vi "Handle Connections Value Change.vi"(4 "State":string, 5 "Alias Mappings":T4[](array[typedef]), 6 "Possible Connections":T3(array[cluster])=[{"Resource"="", "Possible Connections"=[]}, {"Resource"="", "Possible Connections"=[]}], 7 "Alias Mappings by Module":T1(array[cluster]), 8 "error in (no error)":errorcluster, 9 "OldVal":T5[](array[typedef]), 10 "NewVal":T5[](array[typedef]), 11 "Routing Channel Ref in":T6 format="%.0x") -> (0 "error out":errorcluster, 3 "Routing Channel Ref out":T6 format="%.0x")   [LabVIEW 2017, in "Routing and Faulting System Explorer.lvlib"]
uses:
  Routing and Faulting System Explorer.lvlib
  <vilib>/NI Veristand/Custom Device API/Custom Device Item Ref.ctl
  Connection Row.ctl
  Shared/Alias Mapping.ctl
  Shared/Routing and Faulting Hardware API/Types/Possible Connections for Endpoint.ctl
  e32bcdcd-e61b-4a24-afe7-32b08c6141fc.vi
  Scripting/Routing and Faulting Scripting.lvlib
  <vilib>/NI VeriStand/Custom Device API/Custom Device API.lvlib
  Shared/Routing and Faulting Shared.lvlib
  Shared/Routing and Faulting Hardware API/Routing and Faulting Hardware API.lvlib
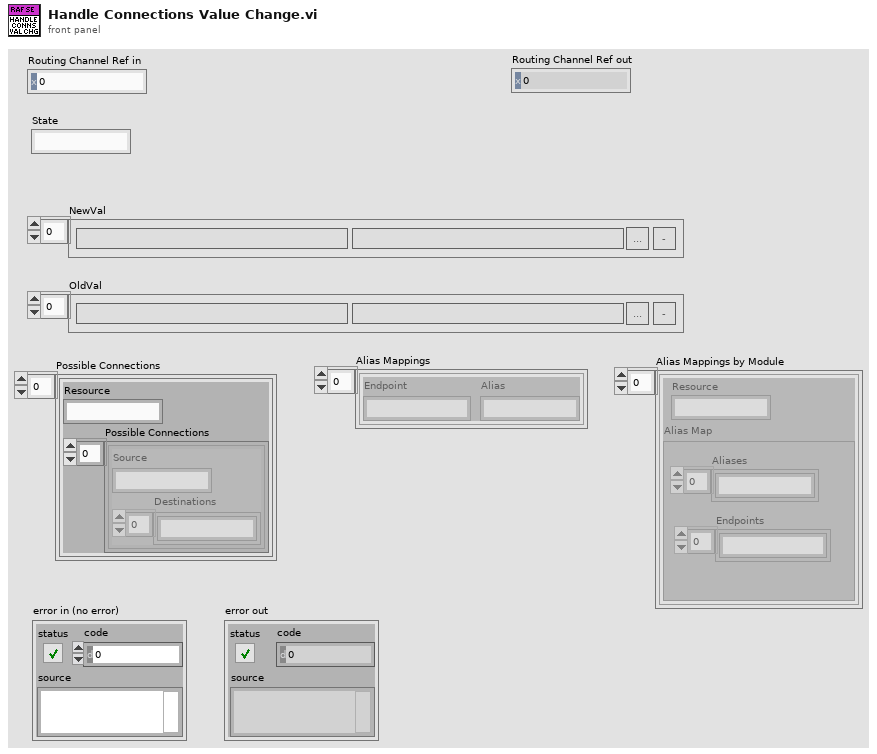
[diagram p1: front panel]
types:
  T1 = cluster{"Resource":string, "Alias Map":cluster{"Aliases":string[], "Endpoints":string[]}}[]
  T2 = typedef "Routing and Faulting Hardware API.lvlib/Possible Connections for Endpoint.ctl" = cluster{"Source":string, "Destinations":string[]}
  T3 = cluster{"Resource":string, "Possible Connections":T2[]}[]
  T4 = typedef "Routing and Faulting Shared.lvlib/Alias Mapping.ctl" = cluster{"Endpoint":string, "Alias":string}
  T5 = typedef "Routing and Faulting System Explorer.lvlib/Connection Row.ctl" = cluster{"Source":string, "Destination":string, "Edit":bool, "Remove":bool}
  T6 = typedef "Custom Device API.lvlib/Custom Device Item Ref.ctl" = u64
  T7 = cluster{"Source":bool, "Destination":bool, "Edit":bool, "Remove":bool}
  T8 = typedef "Routing and Faulting Shared.lvlib/Connection.ctl" = cluster{"Module":string, "Source":string, "Destination":string}
  T9 = typedef "Routing and Faulting Shared.lvlib/Routing State.ctl" = cluster{"Name":string, "Description":string, "Value":i32, "Connection List":T8[]}
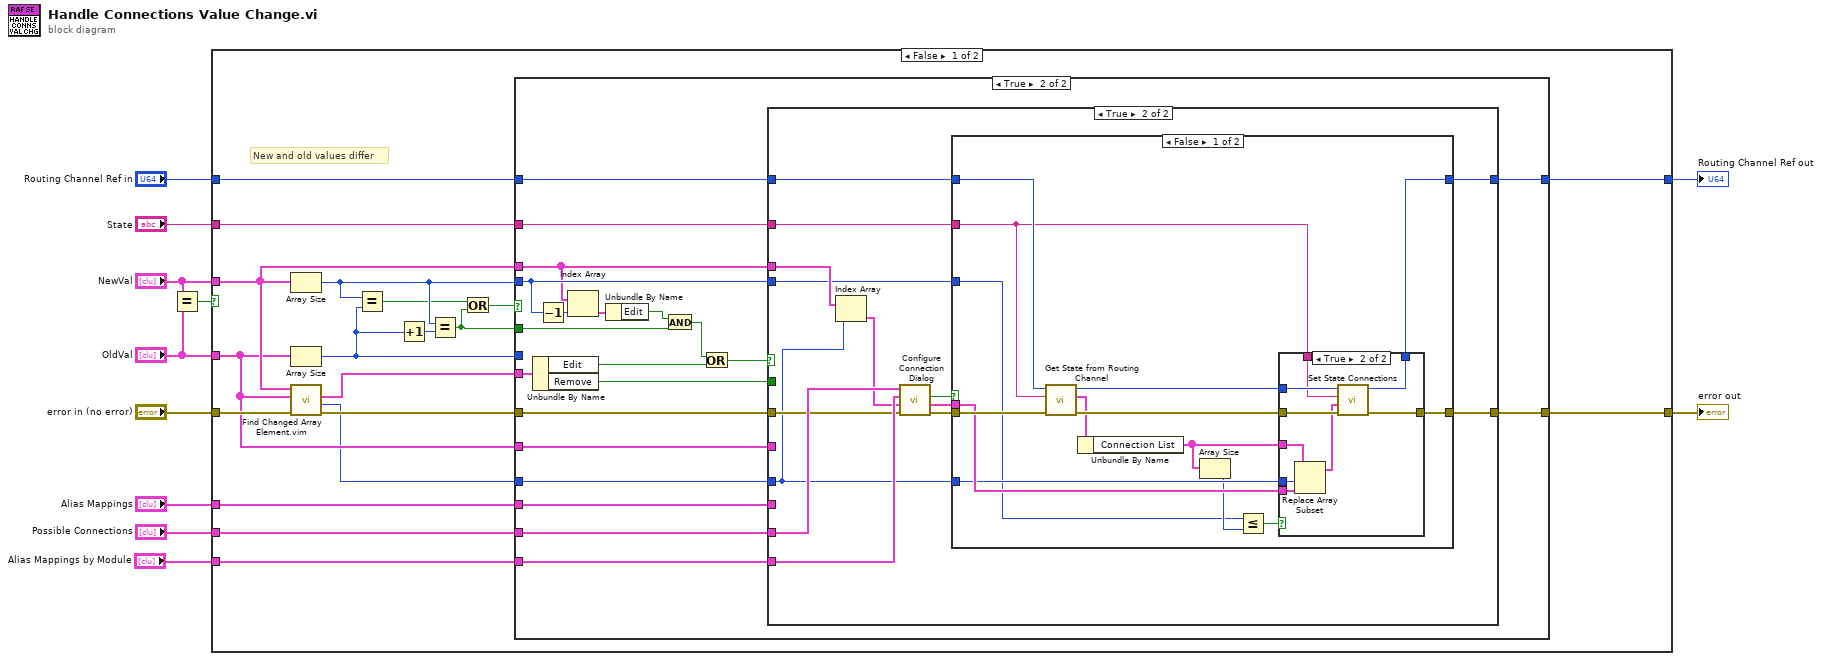
[diagram p0: block diagram]
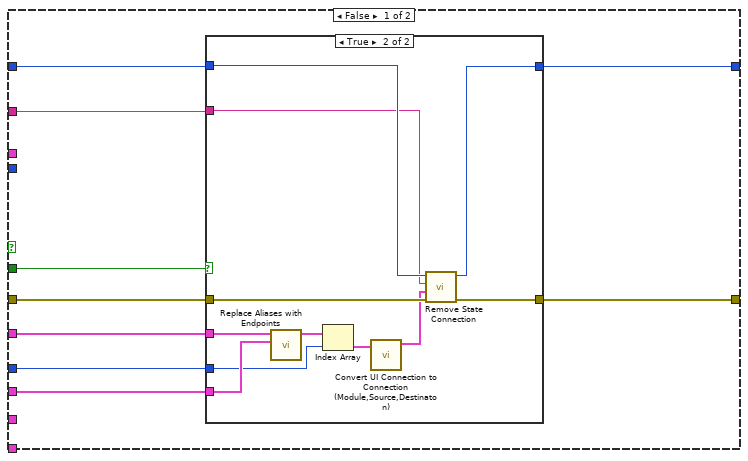
[diagram p3: hidden frame]
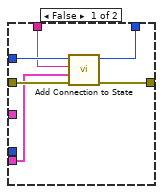
[diagram p5: hidden frame]
diagram:
  n1 = Equal?(x="NewVal", y="OldVal") -> (x = y?=w7:bool)
  n2 = case shown="False" w7 {
    tunnel: "error in (no error)" -> [w30 w121]
    tunnel: "Routing Channel Ref in" -> [w28 w122]
    tunnel: "NewVal" -> [w27 _]
    tunnel: "OldVal" -> [w26 _]
    tunnel: [w24 w121] -> w9
    tunnel: [w23 w122] -> w8
    tunnel: "State" -> [w21 _]
    tunnel: "Alias Mappings" -> [w20 _]
    tunnel: "Possible Connections" -> [w19 _]
    tunnel: "Alias Mappings by Module" -> [w18 _]
    frame False {
      # "New and old values differ"
      n3 = Array Size(array=w27) -> (size(s)=w15:i32)
      n4 = Array Size(array=w26) -> (size(s)=w17:i32)
      n5 = call "Find Changed Array Element.vim"("error in (no error)"=w30, "OldVal"=w26, "NewVal"=w27) -> ("error out"=w25:errorcluster, "Array Index"=w22:i32, "Element Changed"=w29:T7)  [unwired: 6 in]
      n6 = Equal?(x=w15, y=w17) -> (x = y?=w13:bool)
      n7 = Increment(x=w17) -> (x+1=w16:i32)
      n8 = Equal?(x=w15, y=w16) -> (x = y?=w12:bool)
      n9 = Or(x=w13, y=w12) -> (x .or. y?=w14:bool)
      n10 = case shown="True" w14 {
        tunnel: w22 -> [_ w47]
        tunnel: w29 -> [_ w53]
        tunnel: w15 -> [_ w39]
        tunnel: w17 -> [_ _]
        tunnel: w28 -> [w32 w51]
        tunnel: w27 -> [_ w37]
        tunnel: w26 -> [_ w52]
        tunnel: w25 -> [w31 w48]
        tunnel: [w31 w50] -> w24
        tunnel: [w32 w49] -> w23
        tunnel: w21 -> [_ w46]
        tunnel: w20 -> [_ w45]
        tunnel: w19 -> [_ w44]
        tunnel: w18 -> [_ w43]
        tunnel: w12 -> [_ w34]
        frame False {
          # "This case can happen if items are inserted or removed from the array\nshortcut menu during runtime. This is a lot of extra code to handle,\nso the shortcut menu for the Connections array is\ncurrently disabled to prevent this code path.\nIf the shortcut menu is ever re-enabled, code for handling add/remove\nshould go in this case."
        }
        frame True {
          n11 = Unbundle By Name(w53) -> ("Edit"=w42:bool, "Remove"=w41:bool)
          n12 = Decrement(x=w39) -> (x-1=w38:i32)
          n13 = Index Array(array=w37, index=w38) -> (element=w36:T5)
          n14 = Unbundle By Name(w36) -> ("Edit"=w35:bool)
          n15 = And(x=w35, y=w34) -> (x .and. y?=w33:bool)
          n16 = Or(x=w33, y=w42) -> (x .or. y?=w40:bool)
          n17 = case shown="True" w40 {
            tunnel: w52 -> [w62 _]
            tunnel: w51 -> [w61 w89]
            tunnel: [w60 w80] -> w50
            tunnel: [w59 w79] -> w49
            tunnel: w48 -> [w58 w85]
            tunnel: w37 -> [_ w77]
            tunnel: w47 -> [w57 w81]
            tunnel: w46 -> [w56 w78]
            tunnel: w45 -> [w55 _]
            tunnel: w41 -> [w54 _]
            tunnel: w44 -> [_ w88]
            tunnel: w43 -> [_ w87]
            tunnel: w39 -> [_ w76]
            frame False {
              n18 = case shown="True" w54 {
                tunnel: w57 -> [_ w65]
                tunnel: w61 -> [w64 w73]
                tunnel: w62 -> [_ w75]
                tunnel: w58 -> [w63 w72]
                tunnel: [w63 w67] -> w60
                tunnel: [w64 w71] -> w59
                tunnel: w56 -> [_ w66]
                tunnel: w55 -> [_ w69]
                frame False {
                }
                frame True {
                  n19 = call "Replace Aliases with Endpoints.vi"("Alias Mappings"=w69, "UI Connections List in"=w75) -> ("UI Connections List out"=w70:T5[])  [unwired: 9 in]
                  n20 = Index Array(array=w70, index=w65) -> (element=w74:T5)
                  n21 = call "Convert UI Connection to Connection (Module,Source,Destinaton).vi"("Connection"=w74) -> ("Connection (Module,Source,Destinaton)"=w68:T8)  [unwired: 10 in]
                  n22 = call "Remove State Connection.vi"("error in (no error)"=w72, "Connection"=w68, "State"=w66, "Channel Ref in"=w73) -> ("error out"=w67:errorcluster, "Channel Ref out"=w71:T6)  [unwired: 6 in]
                }
              }
            }
            frame True {
              n23 = Index Array(array=w77, index=w81) -> (element=w86:T5)
              n24 = call "Configure Connection Dialog.vi"("error in (no error)"=w85, "Current Connection"=w86, "Alias Mappings by Module"=w87, "Possible Connections"=w88) -> ("error out"=w84:errorcluster, "Connection (R,S,D)"=w83:T8, "Canceled?"=w82:bool)  [unwired: 5 in]
              n25 = case shown="False" w82 {
                tunnel: w89 -> [w102 w119]
                tunnel: w83 -> [w98 _]
                tunnel: w84 -> [w101 w120]
                tunnel: [w99 w120] -> w80
                tunnel: w81 -> [w96 _]
                tunnel: [w95 w119] -> w79
                tunnel: w78 -> [w94 _]
                tunnel: w76 -> [w90 _]
                frame False {
                  n26 = call "Get State from Routing Channel.vi"("error in (no error)"=w101, "State"=w94, "Channel Ref in"=w102) -> ("error out"=w100:errorcluster, "State and Connections"=w97:T9, "Channel Ref out"=w103:T6)  [unwired: 6 in]
                  n27 = Unbundle By Name(w97) -> ("Connection List"=w93:T8[])
                  n28 = Array Size(array=w93) -> (size(s)=w92:i32)
                  n29 = Less Or Equal?(x=w90, y=w92) -> (x <= y?=w91:bool)
                  n30 = case shown="True" w91 {
                    tunnel: w103 -> [w109 w118]
                    tunnel: w100 -> [w108 w117]
                    tunnel: [w106 w116] -> w99
                    tunnel: w98 -> [w105 w115]
                    tunnel: w96 -> [_ w114]
                    tunnel: [w107 w112] -> w95
                    tunnel: w94 -> [w104 w111]
                    tunnel: w93 -> [_ w110]
                    frame False {
                      n31 = call "Add Connection to State.vi"("error in (no error)"=w108, "Connection"=w105, "State"=w104, "Channel Ref in"=w109) -> ("error out"=w106:errorcluster, "Channel Ref out"=w107:T6)  [unwired: 6 in]
                    }
                    frame True {
                      n32 = Replace Array Subset(array=w110, new element=w115, index=w114) -> (w113:T8[])
                      n33 = call "Set State Connections.vi"("error in (no error)"=w117, "Connection List"=w113, "State"=w111, "Channel Ref in"=w118) -> ("error out"=w116:errorcluster, "Channel Ref out"=w112:T6)  [unwired: 6 in]
                    }
                  }
                }
                frame True {
                }
              }
            }
          }
        }
      }
    }
    frame True {
      # "New and old values are the same. Do nothing"
    }
  }
  "Routing Channel Ref out" <- w8
  "error out" <- w9
